vi "Example 01 Picture Ring Static.vi"() -> ()   [LabVIEW 2019, in "Grassfire 2D.lvclass"]
uses:
  Grassfire 2D.lvclass
  Selection--array.ctl
  Selection--picture ring.ctl
  Direction--enum.ctl
  Solution Node--cluster.ctl
  Solution--picture ring.ctl
panel:
  out "ms":u32
  out "Solution Grid":T1[][](array[typedef])
  out "Directions":T3[](array[typedef])
  in  "Selection Grid":T4
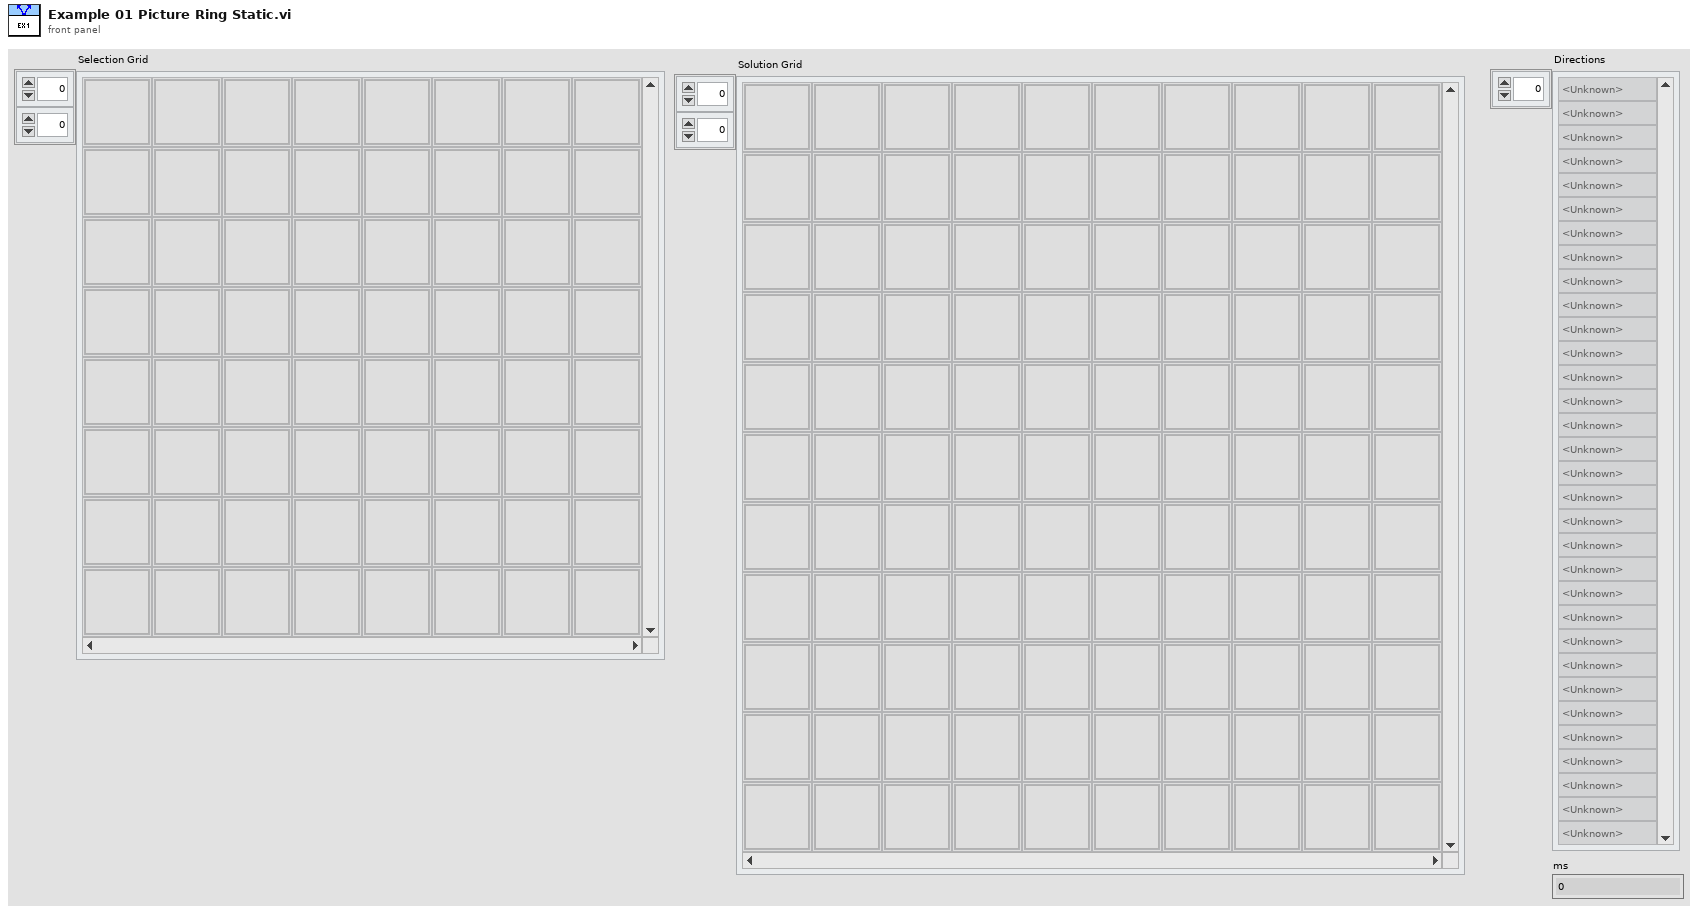
[diagram p1: front panel]
types:
  T1 = typedef "Grassfire 2D.lvclass/Solution Node--cluster.ctl" = cluster{"Picture":T2, "Value":string}
  T2 = typedef "Grassfire 2D.lvclass/Solution--picture ring.ctl" = i64
  T3 = typedef "Grassfire 2D.lvclass/Direction--enum.ctl" = enum16{"<Unknown>", "Right", "Down", "Left", "Up"}
  T4 = typedef "Grassfire 2D.lvclass/Selection--array.ctl" = cluster{"Grid Value":T5}[][]
  T5 = typedef "Grassfire 2D.lvclass/Selection--picture ring.ctl" = i64
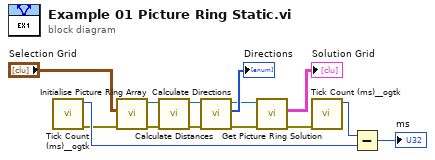
[diagram p0: block diagram]
diagram:
  n1 = call <userlib>:"Tick Count (ms)__ogtk.vi"() -> ("error out"=w3:errorcluster, "millisecond timer value"=w4:u32)  [unwired: 10 in]
  n2 = call "Initialise Picture Ring Array.vi"("error in (no error)"=w3, "Selection Grid"="Selection Grid") -> ("error out"=w8:errorcluster, "Grassfire 2D out"=w13:refnum<class "Grassfire 2D.lvclass">)  [unwired: 7 in, 1 out]
  n3 = call-dynamic "Calculate Distances.vi"("error in (no error)"=w8, "Grassfire 2D In"=w13) -> ("error out"=w7:errorcluster, "Grassfire 2D Out"=w12:refnum<class "Grassfire 2D.lvclass">)  [unwired: 8 in]
  n4 = call-dynamic "Calculate Directions.vi"("error in (no error)"=w7, "Grassfire 2D In"=w12) -> ("error out"=w6:errorcluster, "Directions"=→"Directions":T3[], "Grassfire 2D Out"=w10:refnum<class "Grassfire 2D.lvclass">)  [unwired: 7 in]
  n5 = call "Get Picture Ring Solution.vi"("error in (no error)"=w6, "Grassfire 2D In"=w10) -> ("error out"=w2:errorcluster, "Array"=→"Solution Grid":T1[][])  [unwired: 7 in, 1 out]
  n6 = call <userlib>:"Tick Count (ms)__ogtk.vi"("error in (no error)"=w2) -> ("millisecond timer value"=w5:u32)  [unwired: 9 in, 1 out]
  n7 = Subtract(x=w5, y=w4) -> (x-y=→"ms":u32)
